vi "Write PID gains.vi"(8 "error in (no error)":errorcluster, 10 "PID gains":cluster{"P":dbl, "I":dbl, "D":dbl}={"P"=1.0, "I"=0.01, "D"=0.0}, 11 "Plant in":refnum<class "Plant.lvclass">) -> (0 "error out":errorcluster, 3 "Plant out":refnum<class "Plant.lvclass">)   [LabVIEW 2023, in "Plant.lvlib" / "Plant.lvclass"]
uses:
  Plant.lvclass
  Plant.lvclass/Plant.ctl
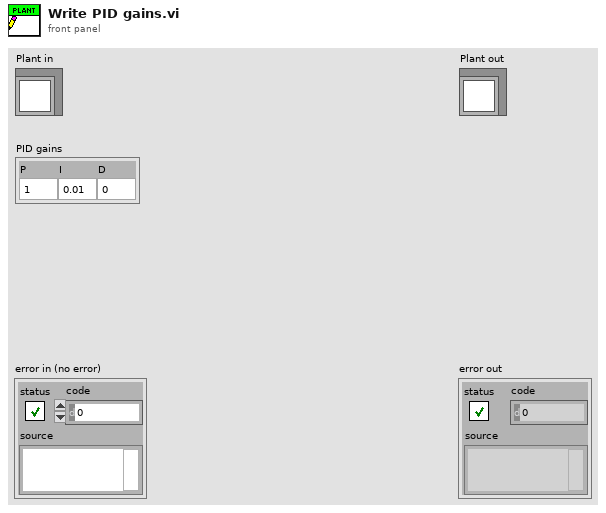
[diagram p1: front panel]
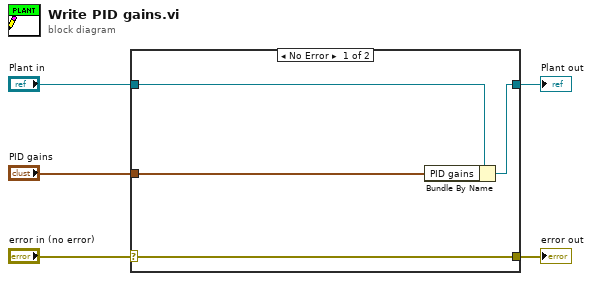
[diagram p0: block diagram]
diagram:
  n1 = case shown="No Error" "error in (no error)" {
    selector: "error in (no error)" -> [w9 w10]
    tunnel: [w9 w10] -> w4
    tunnel: [w7 w11] -> w2
    tunnel: "Plant in" -> [w8 w11]
    tunnel: "PID gains" -> [w6 _]
    frame No Error {
      n2 = Bundle By Name(cluster=w8, "PID gains"=w6) -> (w7:refnum<class "Plant.lvclass">)
    }
    frame Error {
    }
  }
  "error out" <- w4
  "Plant out" <- w2
